vi "SAOMM-ProcImageParser.vi"(7 "ProcessedData":u8[](array[numeric])=array[44904 elements]) -> (4 "ImageBuffer":u16[][](graph), 6 "GrayLevels":u8[][](graph), 10 "MaskObjet":u8[][](graph), 12 "GeneralProperties":T3, 13 "ROIProperties":T1, 14 "ProcessedProperties":T2 {"Centroide Y" format="%.3f"; "Centroide X" format="%.3f"; "SNR" format="%.3f"; "Flux" format="%.3f"; "Seuil du masque" format="%.3f"}, 15 "MaskSeuil":u8[][](graph))   [LabVIEW 2011]
uses:
  Polymorphics/Num2littleEndian(U16).vi
panel:
  out "size(s)":i32
  out "Height":i32
  out "Width":i32
  out "ImageLen":i32
  out "BufferLen":i32
  out "ImagesIndex":i32
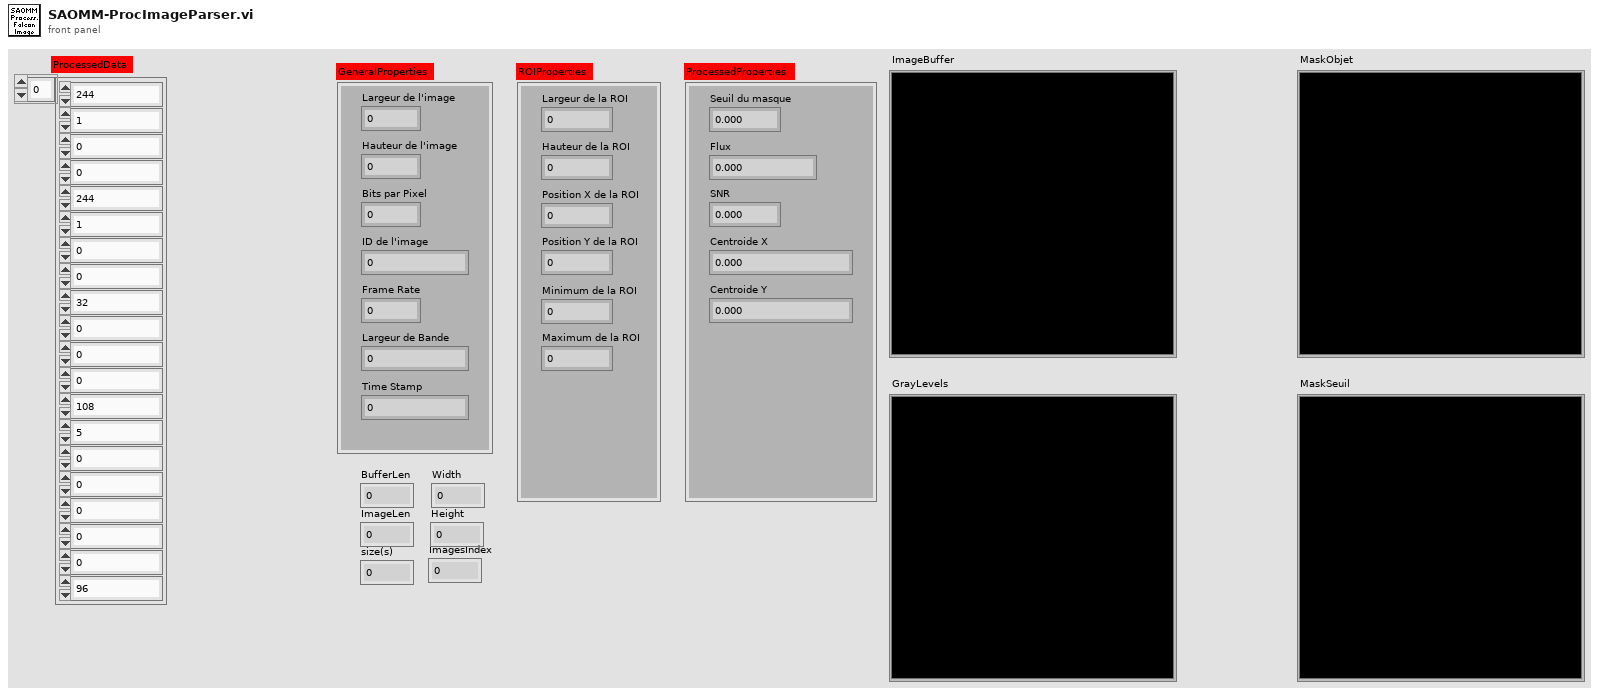
[diagram p1: front panel]
types:
  T1 = cluster{"Largeur de la ROI":u16, "Hauteur de la ROI":u16, "Position X de la ROI":u16, "Position Y de la ROI":u16, "Minimum de la ROI":u32, "Maximum de la ROI":u32}
  T2 = cluster{"Seuil du masque":dbl, "Flux":dbl, "SNR":dbl, "Centroide X":dbl, "Centroide Y":dbl}
  T3 = cluster{"Largeur de l'image":dbl, "Hauteur de l'image":dbl, "Bits par Pixel":dbl, "ID de l'image":u32, "Frame Rate":dbl, "Largeur de Bande":dbl, "Time Stamp":u64}
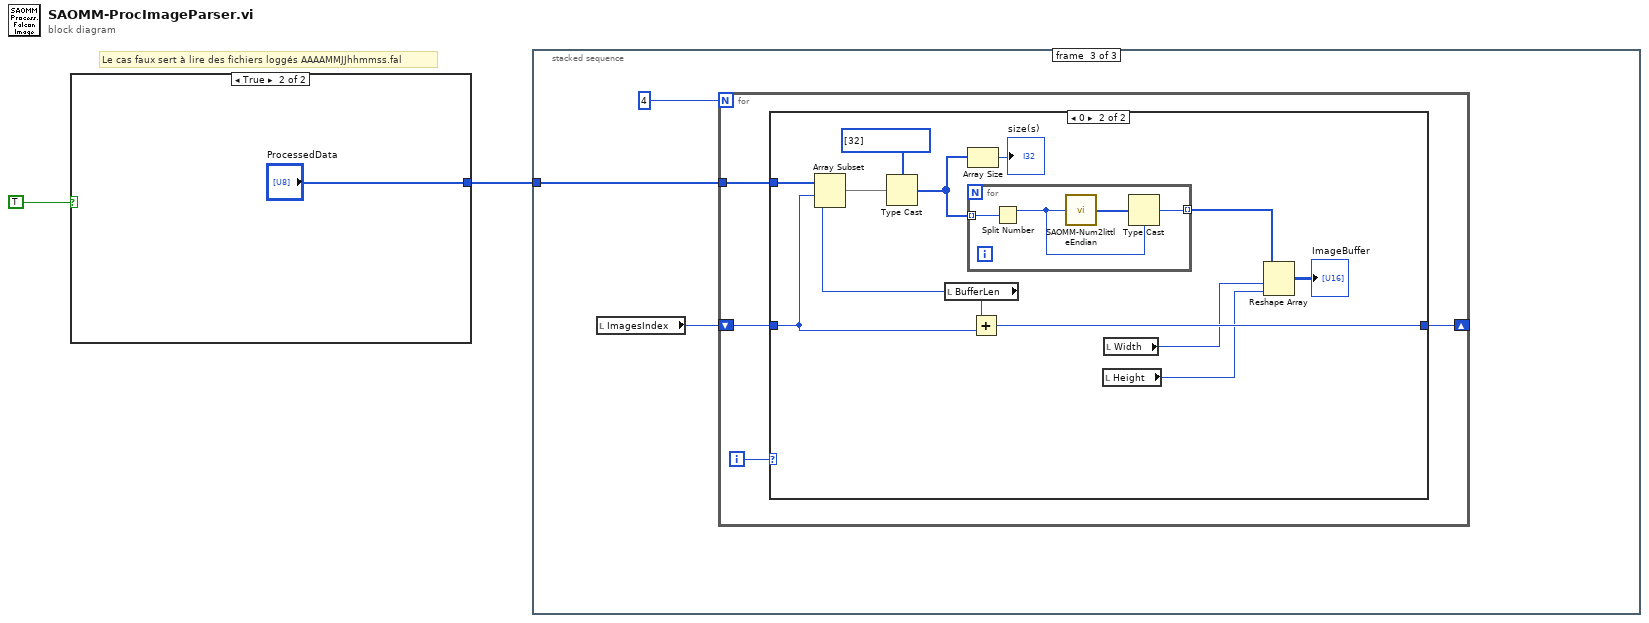
[diagram p0: block diagram]
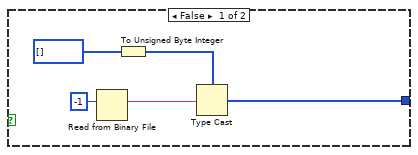
[diagram p2: hidden frame]
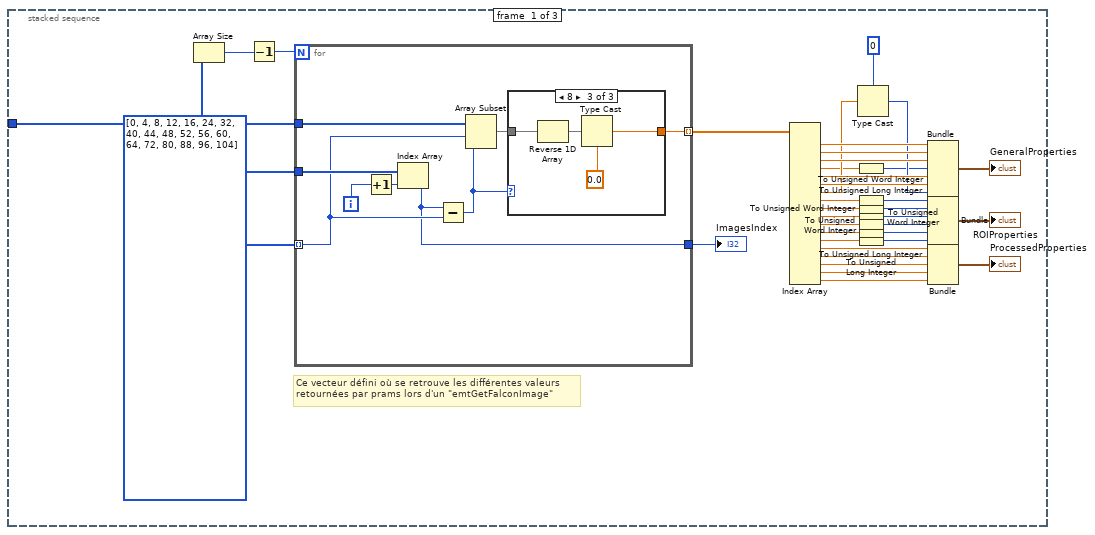
[diagram p3: hidden frame]
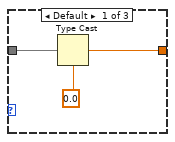
[diagram p4: hidden frame]
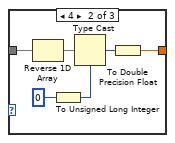
[diagram p5: hidden frame]
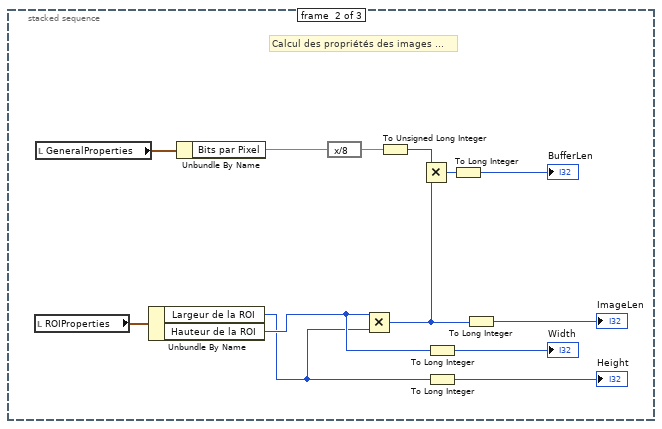
[diagram p6: hidden frame]
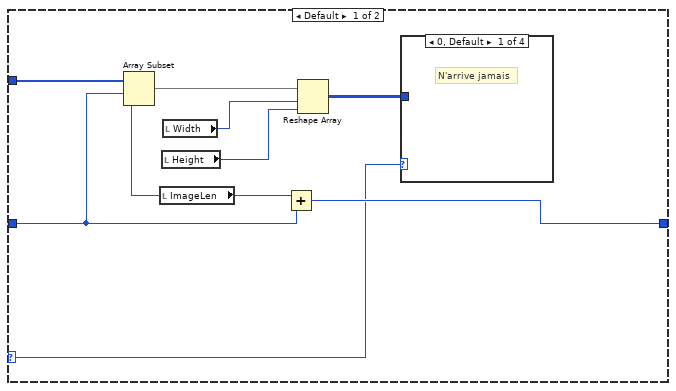
[diagram p7: hidden frame]
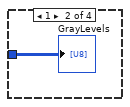
[diagram p8: hidden frame]
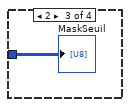
[diagram p9: hidden frame]
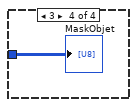
[diagram p10: hidden frame]
diagram:
  # "Le cas faux sert à lire des fichiers loggés AAAAMMJJhhmmss.fal"
  n1 = case shown="True" TRUE ("À remettre en constante ...") {
    tunnel: [w3 "ProcessedData"] -> w1
    frame False {
      n2 = Read from Binary File(10:-1 ("count (1)")) -> (2:w5:string)  [unwired: 5 in, 3 out]
      n3 = To Unsigned Byte Integer(number=u8[] []) -> (unsigned 8bit integer=w4:u8[])
      n4 = Type Cast(type=w4, x=w5) -> (*(type *) &x=w3:u8[])
    }
    frame True {
    }
  }
  n5 = stacked-sequence {
    tunnel: w1 -> [w44 _ w82]
    frame #0 {
      w24 = i32[] [0, 4, 8, 12, 16, 24, 32, 40, 44, 48, 52, 56, 60, 64, 72, 80, 88, 96, 104] ("ValuesIndex")
      # "Ce vecteur défini où se retrouve les différentes valeurs\nretournées par prams lors d'un \"emtGetFalconImage\""
      n6 = Array Size(array=w24) -> (size(s)=w41:i32)
      n7 = Decrement(x=w41) -> (x-1=w42:i32)
      n8 = for {
        N: w42 -> [_]
        tunnel: w44 -> [w53]
        tunnel: w24 -> [w46] mode=indexing
        tunnel: w24 -> [w50]
        tunnel: [w47] -> w43 mode=indexing
        tunnel: [w45] -> w20
        i -> [w51]
        n9 = Increment(x=w51) -> (x+1=w52:i32)
        n10 = Index Array(array=w50, index=w52) -> (element=w45:i32)
        n11 = Subtract(x=w45, y=w46) -> (x-y=w48:i32)
        n12 = Array Subset(array=w53, index=w46, length=w48) -> (w49:u8[])
        n13 = case shown="8" w48 {
          tunnel: w49 -> [w56 w58 w63]
          tunnel: [w55 w59 w64] -> w47
          frame Default {
            n14 = Type Cast(type=0.0, x=w56) -> (*(type *) &x=w55:dbl)
          }
          frame 4 {
            n15 = Reverse 1D Array(array=w58) -> (reversed array=w57:u8[])
            n16 = To Unsigned Long Integer(number=0) -> (unsigned 32bit integer=w61:u32)
            n17 = Type Cast(type=w61, x=w57) -> (*(type *) &x=w60:u32)
            n18 = To Double Precision Float(number=w60) -> (double precision float=w59:dbl)
          }
          frame 8 {
            n19 = Reverse 1D Array(array=w63) -> (reversed array=w66:u8[])
            n20 = Type Cast(type=0.0, x=w66) -> (*(type *) &x=w64:dbl)
          }
        }
      }
      "ImagesIndex" <- w20
      n21 = Index Array(array=w43) -> (element #1=w30:dbl, element #2=w29:dbl, element #3=w28:dbl, element #4=w14:dbl, element #5=w27:dbl, element #6=w26:dbl, element #7=w23:dbl, element #8=w34:dbl, element #9=w33:dbl, element #10=w32:dbl, element #11=w31:dbl, element #12=w12:dbl, element #13=w10:dbl, element #14=w40:dbl, element #15=w39:dbl, element #16=w38:dbl, element #17=w37:dbl, element #18=w36:dbl)  [unwired: 18 in]
      n22 = To Unsigned Long Integer(number=w14) -> (unsigned 32bit integer=w15:u32)
      n23 = To Unsigned Word Integer(number=w34) -> (unsigned 16bit integer=w19:u16)
      n24 = To Unsigned Word Integer(number=w33) -> (unsigned 16bit integer=w18:u16)
      n25 = To Unsigned Word Integer(number=w32) -> (unsigned 16bit integer=w17:u16)
      n26 = To Unsigned Word Integer(number=w31) -> (unsigned 16bit integer=w16:u16)
      n27 = To Unsigned Long Integer(number=w12) -> (unsigned 32bit integer=w11:u32)
      n28 = To Unsigned Long Integer(number=w10) -> (unsigned 32bit integer=w9:u32)
      n29 = Type Cast(type=u64 0, x=w23) -> (*(type *) &x=w22:u64)
      n30 = Bundle(w30, w29, w28, w15, w27, w26, w22) -> (→"GeneralProperties":cluster{dbl, dbl, dbl, u32, dbl, dbl, u64})  [unwired: 1 in]
      n31 = Bundle(w19, w18, w17, w16, w11, w9) -> (→"ROIProperties":cluster{u16, u16, u16, u16, u32, u32})  [unwired: 1 in]
      n32 = Bundle(w40, w39, w38, w37, w36) -> (→"ProcessedProperties":cluster{dbl, dbl, dbl, dbl, dbl})  [unwired: 1 in]
    }
    frame #1 {
      # "Calcul des propriétés des images ..."
      n33 = local read "ROIProperties"() -> (w79:T1)
      n34 = local read "GeneralProperties"() -> (w78:T3)
      n35 = Unbundle By Name(w79) -> ("Largeur de la ROI"=w67:u16, "Hauteur de la ROI"=w68:u16)
      n36 = Unbundle By Name(w78) -> ("Bits par Pixel"=w77:dbl)
      n37 = expression code="x/8"(w77) -> (w72:dbl)
      n38 = Multiply(x=w68, y=w67) -> (x*y=w76:u16)
      n39 = To Unsigned Long Integer(number=w72) -> (unsigned 32bit integer=w71:u32)
      n40 = Multiply(x=w71, y=w76) -> (x*y=w70:u32)
      n41 = To Long Integer(number=w68) -> (32bit integer=→"Width":i32)
      n42 = To Long Integer(number=w67) -> (32bit integer=→"Height":i32)
      n43 = To Long Integer(number=w70) -> (32bit integer=→"BufferLen":i32)
      n44 = To Long Integer(number=w76) -> (32bit integer=→"ImageLen":i32)
    }
    frame #2 {
      n45 = local read "ImagesIndex"() -> (w81:i32)
      n46 = for {
        N: 4 -> [_]
        tunnel: w82 -> [w84]
        shift-right: [w83] -> _
        shift-left: w81 -> [w85]
        i -> [w86]
        n47 = case shown="0" w86 {
          selector: w86 -> [w88 _]
          tunnel: w85 -> [w92 w110]
          tunnel: w84 -> [w94 w104]
          tunnel: [w95 w108] -> w83
          frame Default {
            n48 = local read "ImageLen"() -> (w93:i32)
            n49 = Array Subset(array=w94, index=w92, length=w93) -> (w89:u8[])
            n50 = local read "Height"() -> (w90:i32)
            n51 = local read "Width"() -> (w91:i32)
            n52 = Add(x=w93, y=w92) -> (x+y=w95:i32)
            n53 = Reshape Array(w89, w91, w90) -> (w87:u8[][])
            n54 = case shown="0, Default" w88 {
              tunnel: w87 -> [_ w96 w97 w98]
              frame 0, Default {
                # "N'arrive jamais"
              }
              frame 1 {
                "GrayLevels" <- w96
              }
              frame 2 {
                "MaskSeuil" <- w97
              }
              frame 3 {
                "MaskObjet" <- w98
              }
            }
          }
          frame 0 {
            n55 = local read "BufferLen"() -> (w109:i32)
            n56 = Array Subset(array=w104, index=w110, length=w109) -> (w103:u8[])
            n57 = Type Cast(type=u32[] [32], x=w103) -> (*(type *) &x=w100:u32[])
            n58 = Array Size(array=w100) -> (size(s)=→"size(s)":i32)
            n59 = for {
              tunnel: w100 -> [w114] mode=indexing
              tunnel: [w113] -> w99 mode=indexing
              n60 = Split Number(x=w114) -> (hi(x)=w111:u16)  [unwired: 1 out]
              n61 = call-poly "SAOMM-Num2littleEndian.vi"("Number"=w111) -> ("LiitleEndianedData"=w112:u8[])  [unwired: 14 in]
              n62 = Type Cast(type=w111, x=w112) -> (*(type *) &x=w113:u16)
            }
            n63 = Add(x=w109, y=w110) -> (x+y=w108:i32)
            n64 = local read "Height"() -> (w106:i32)
            n65 = local read "Width"() -> (w107:i32)
            n66 = Reshape Array(w99, w107, w106) -> (→"ImageBuffer":u16[][])
          }
        }
      }
    }
  }
